vi "Signal Analyzer.vi"() -> ()   [LabVIEW 2014]
panel:
  out "Array":dbl[](array[numeric])
  out "Simulated Frequency":dbl
  in  "Continuous measurements":bool
  in  "Tab Control":enum32{"XY Charts", "Waveform Charts"}(tab)
  out "Phase":cluster{dbl[], dbl[]}(graph)
  out "Impedance":cluster{dbl[], dbl[]}(graph)
  out "Amplitude 3":dynamicdata(graph)
  out "Amplitude":dynamicdata(graph)
  out "Voltage Phase":dynamicdata(graph)
  out "Voltage Frequency":dynamicdata(graph)
  out "Impedance":dynamicdata(graph)
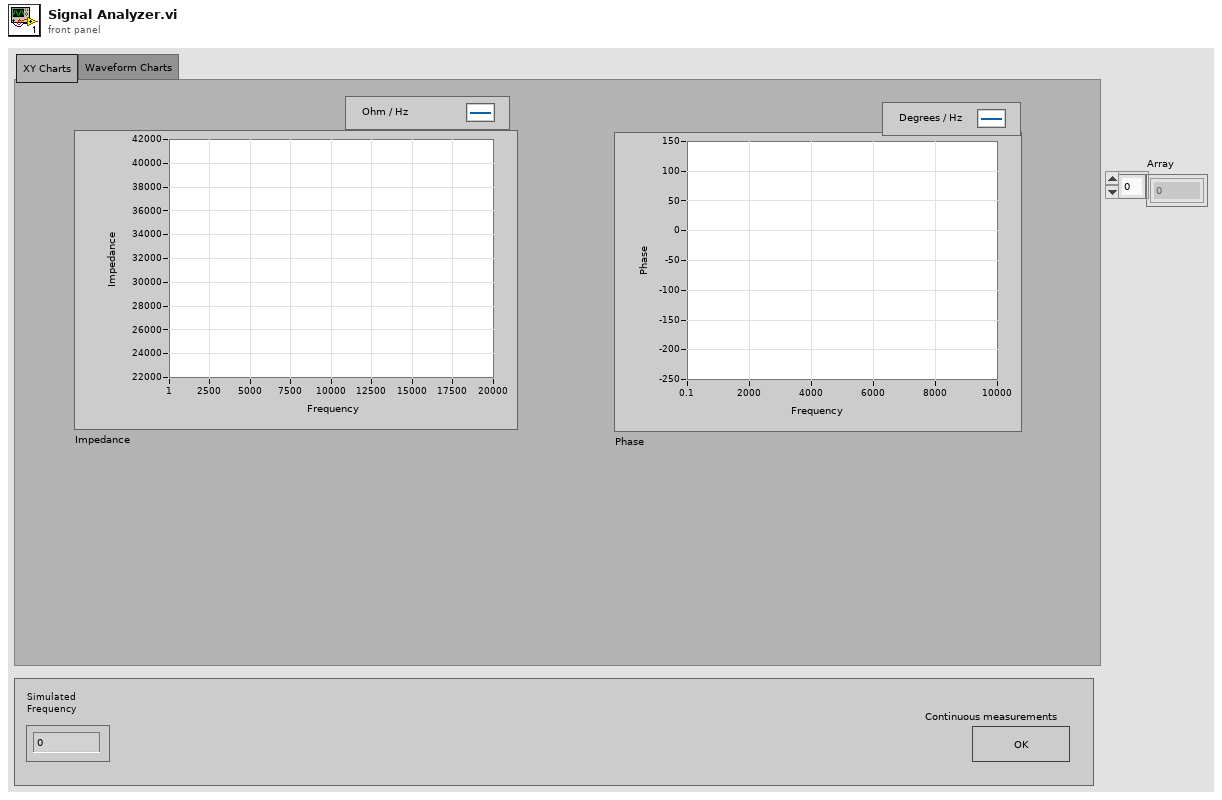
[diagram p1: front panel]
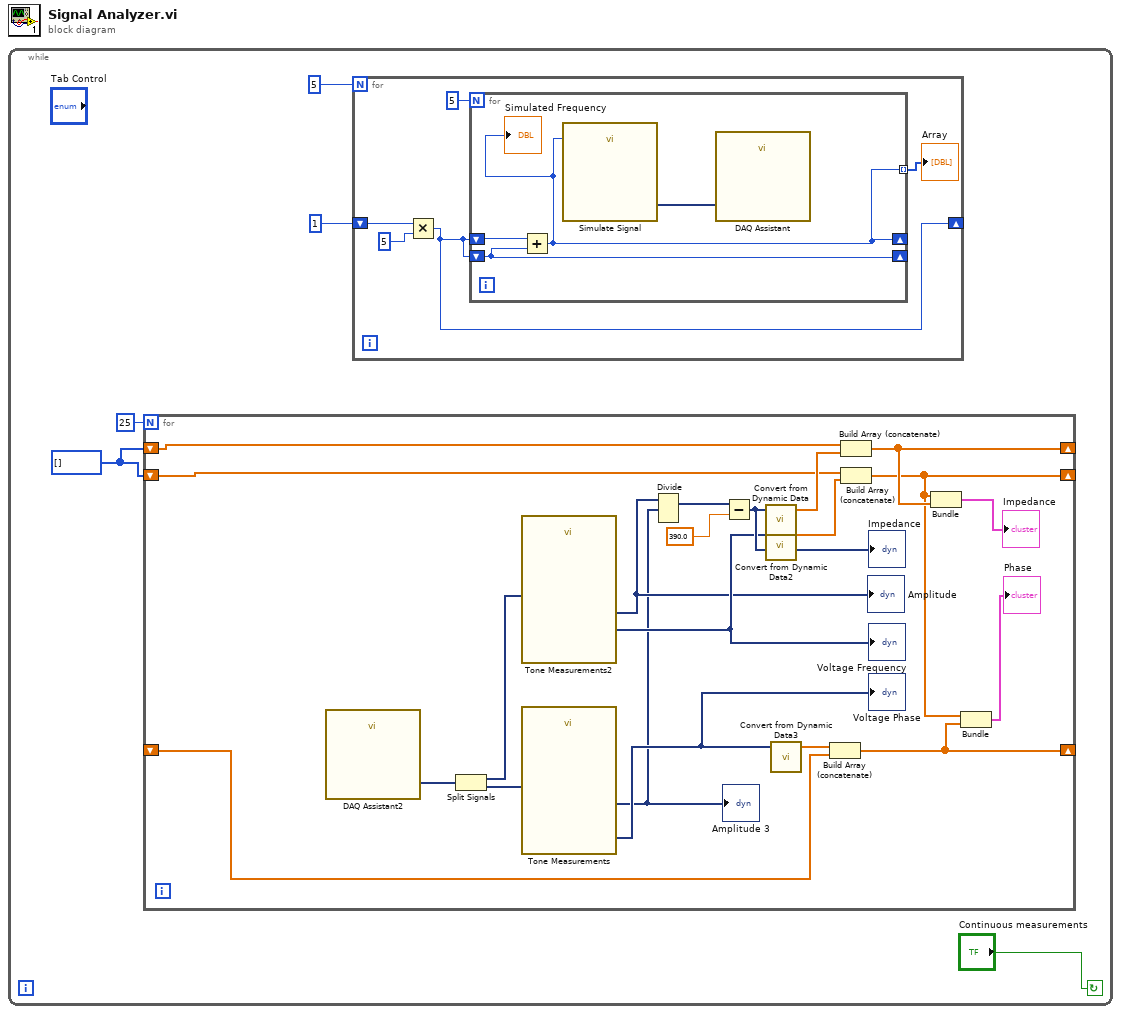
[diagram p0: block diagram]
diagram:
  n1 = while {
    stop <- "Continuous measurements" continue-if-true
    w2 = i32[] []
    n2 = for {
      N: 25 -> [_]
      shift-right: [w17] -> _
      shift-left: w2 -> [w19]
      shift-right: [w10] -> _
      shift-left: w2 -> [w18]
      shift-right: [w11] -> _
      shift-left: _ -> [w12]
      n3 = call "DAQ Assistant2"() -> ("data"=w22:dynamicdata)  [unwired: 16 in, 3 out]
      n4 = Split Signals(w22) -> (w23:dynamicdata, w26:dynamicdata)  [unwired: 2 in]
      n5 = call "Tone Measurements2"("Signals"=w23) -> ("Frequency"=w14:dynamicdata, "Amplitude"=w8:dynamicdata)  [unwired: 7 in, 2 out]
      "Voltage Frequency" <- w14
      "Amplitude" <- w8
      n6 = call "Tone Measurements"("Signals"=w26) -> ("Phase"=w7:dynamicdata, "Amplitude"=w6:dynamicdata)  [unwired: 7 in, 2 out]
      "Voltage Phase" <- w7
      "Amplitude 3" <- w6
      n7 = Divide(1:w6, 2:w8) -> (0:w25:dynamicdata)  [unwired: 1 in, 1 out]
      n8 = Subtract(x=w25, y=390.0) -> (x-y=w15:dynamicdata)
      "Impedance" <- w15
      n9 = call "Convert from Dynamic Data"("Dynamic Data Type"=w15) -> ("Array"=w21:dbl[])  [unwired: 3 in]
      n10 = call "Convert from Dynamic Data2"("Dynamic Data Type"=w14) -> ("Array"=w20:dbl[])  [unwired: 3 in]
      n11 = call "Convert from Dynamic Data3"("Dynamic Data Type"=w7) -> ("Array"=w13:dbl[])  [unwired: 3 in]
      n12 = Build Array (concatenate)(w13, w12) -> (w11:dbl[])
      n13 = Build Array (concatenate)(w19, w21) -> (w17:dbl[])
      n14 = Build Array (concatenate)(w18, w20) -> (w10:dbl[])
      n15 = Bundle(w10, w17) -> (→"Impedance":cluster{dbl[], dbl[]})  [unwired: 1 in]
      n16 = Bundle(w10, w11) -> (→"Phase":cluster{dbl[], dbl[]})  [unwired: 1 in]
    }
    n17 = for {
      N: 5 -> [_]
      shift-right: [w28] -> _
      shift-left: 1 -> [w30]
      n18 = Multiply(x=w30, y=5) -> (x*y=w28:i32)
      n19 = for {
        N: 5 -> [_]
        shift-right: [w32] -> _
        shift-left: w28 -> [w35]
        shift-right: [w34] -> _
        shift-left: w28 -> [w34]
        tunnel: [w32] -> w27 mode=indexing
        n20 = Add(x=w35, y=w34) -> (x+y=w32:i32)
        "Simulated Frequency" <- w32
        n21 = call "Simulate Signal"("Frequency"=w32) -> ("Sine"=w33:dynamicdata)  [unwired: 13 in, 1 out]
        n22 = call "DAQ Assistant"("data"=w33) -> ()  [unwired: 16 in, 3 out]
      }
      "Array" <- w27
    }
  }
